vi "cd-maker.vi"() -> ()   [LabVIEW 2020]
uses:
  <vilib>/Utility/file.llb/Read Delimited Spreadsheet (I64).vi
  <vilib>/Utility/file.llb/Write Delimited Spreadsheet (DBL).vi
  <vilib>/express/express analysis/Spectral/Block/exnSpectralBlock spectral measurements power poly.vi
  <vilib>/express/express analysis/Spectral/Block/exnSpectralBlock spectral measurements power DDT.vi
  <vilib>/express/express analysis/Spectral/XNode/ExpressSpectralMeasurementsBlockNode.xnode
panel:
  in  "Timeout":i32
  out "Waveform Graph 2":dynamicdata(graph)
  out "Waveform Graph":dynamicdata(graph)
  in  "Добавлять точки при\nувеличении размера холста":bool=TRUE
  in  "Очистить полностью":bool
  in  "Стоп":bool
  in  "Путь для загрузки холста карты":path
  in  "Заполнить полностью":bool
  in  "Загрузить холст карты из файла":bool
  in  "Точки холста":bool[][](array[boolean])=[[FALSE, FALSE, FALSE, TRUE, FALSE, TRUE, FALSE, FALSE, FALSE], [FALSE, TRUE, FALSE, FALSE, FALSE, FALSE, FALSE, TRUE, FALSE], [FALSE, FALSE, FALSE, FALSE, FALSE, FALSE, FALSE, FALSE, FALSE], [TRUE, FALSE, FALSE, TRUE, FALSE, TRUE, FALSE, FALSE, TRUE], [FALSE, FALSE, FALSE, FALSE, FALSE, FALSE, FALSE, FALSE, FALSE], [TRUE, FALSE, FALSE, TRUE, FALSE, TRUE, FALSE, FALSE, TRUE], [FALSE, FALSE, FALSE, FALSE, FALSE, FALSE, FALSE, FALSE, FALSE], [FALSE, TRUE, FALSE, FALSE, FALSE, FALSE, FALSE, TRUE, FALSE], [FALSE, FALSE, FALSE, TRUE, FALSE, TRUE, FALSE, FALSE, FALSE]]
  out "Массив I и Q":cluster{"I":sgl, "Q":sgl}[](array[cluster])
  in  "I интервал":sgl=1.0 min=1 step=1
  in  "I смещение":sgl
  in  "Q интервал":sgl=1.0 min=1 step=1
  in  "Q смещение":sgl
  out "Карта":cluster{cluster{"I":sgl, "Q":sgl}[]}[](graph)=[{[{"I"=-1.0, "Q"=4.0}, {"I"=1.0, "Q"=4.0}, {"I"=-3.0, "Q"=3.0}, {"I"=3.0, "Q"=3.0}, {"I"=-4.0, "Q"=1.0}, {"I"=-1.0, "Q"=1.0}, {"I"=1.0, "Q"=1.0}, {"I"=4.0, "Q"=1.0}, {"I"=-4.0, "Q"=-1.0}, {"I"=-1.0, "Q"=-1.0}, {"I"=1.0, "Q"=-1.0}, {"I"=4.0, "Q"=-1.0}, {"I"=-3.0, "Q"=-3.0}, {"I"=3.0, "Q"=-3.0}, {"I"=-1.0, "Q"=-4.0}, {"I"=1.0, "Q"=-4.0}]}, {[{"I"=10.0, "Q"=0.0}, {"I"=-10.0, "Q"=0.0}, {"I"=0.0, "Q"=10.0}, {"I"=0.0, "Q"=-10.0}]}]
  in  "Размер холста":i32(slide)=4 min=1 max=30 step=1 scale=0.0..10.0
  in  "Путь для сохранения холста карты":path
  in  "Сохранить холст карты в файл":bool
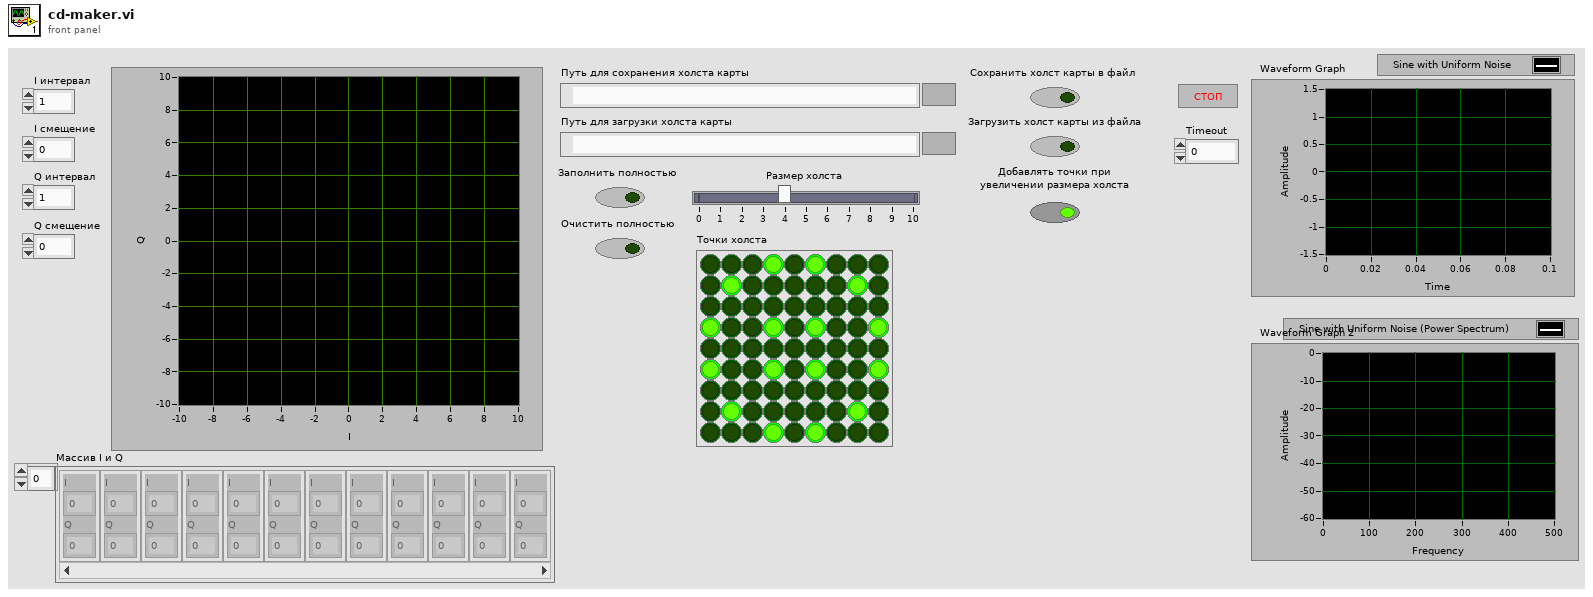
[diagram p1: front panel]
types:
  T1 = cluster{"averaging mode":u16, "weighting mode":u16, "number of averages":u32}
  T2 = cluster{"dB On (F)":bool, "unwrap phase (F)":bool, "convert to degree (F)":bool}
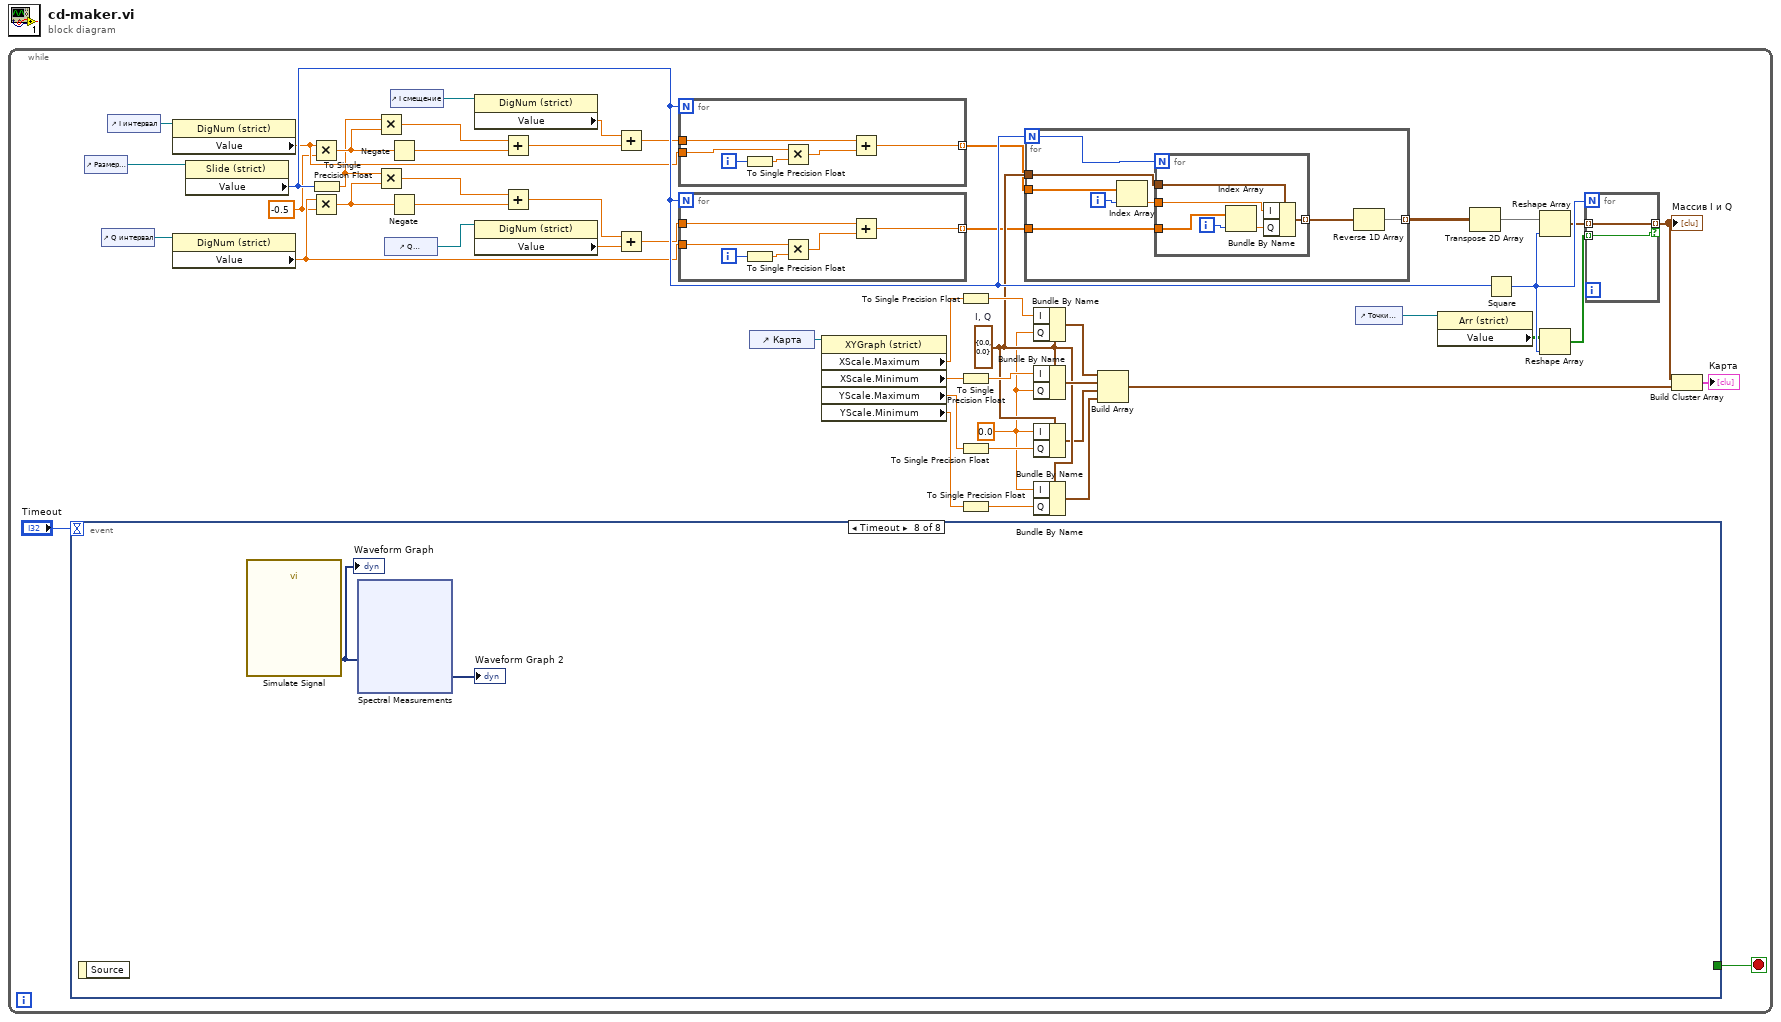
[diagram p0: block diagram]
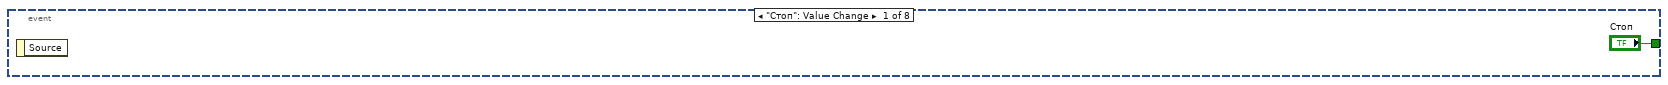
[diagram p2: hidden frame]
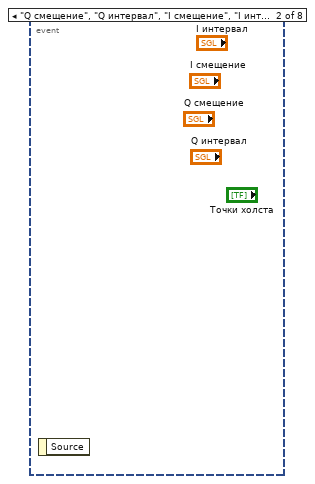
[diagram p3: hidden frame]
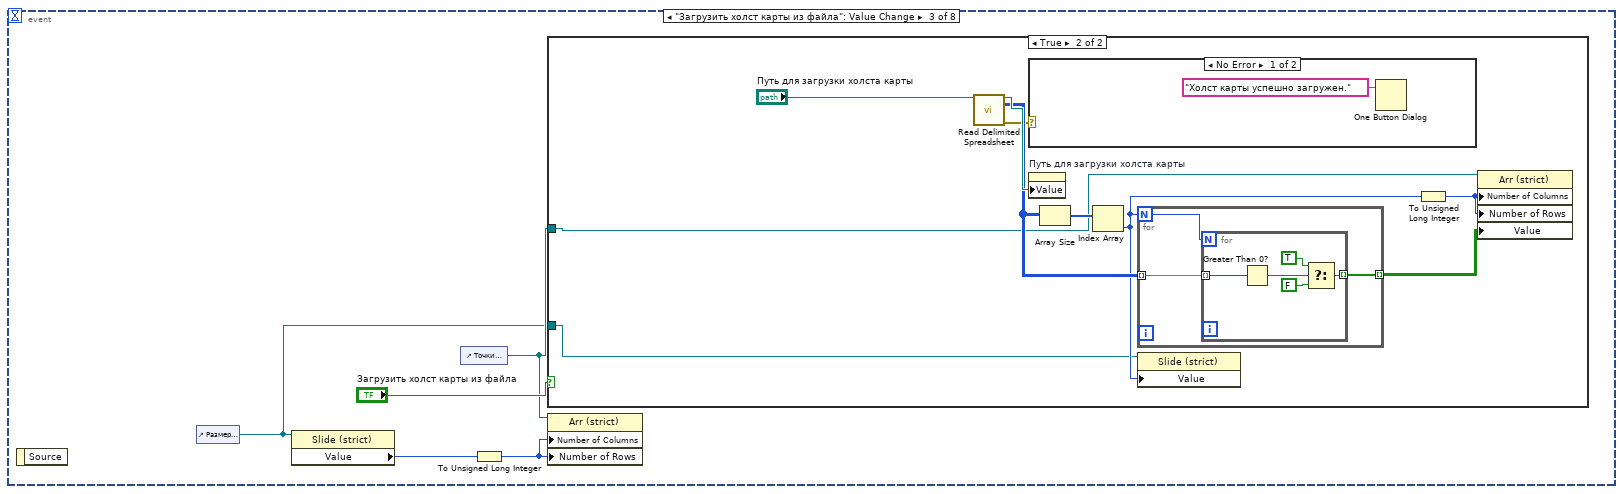
[diagram p4: hidden frame]
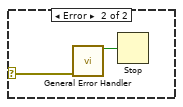
[diagram p6: hidden frame]
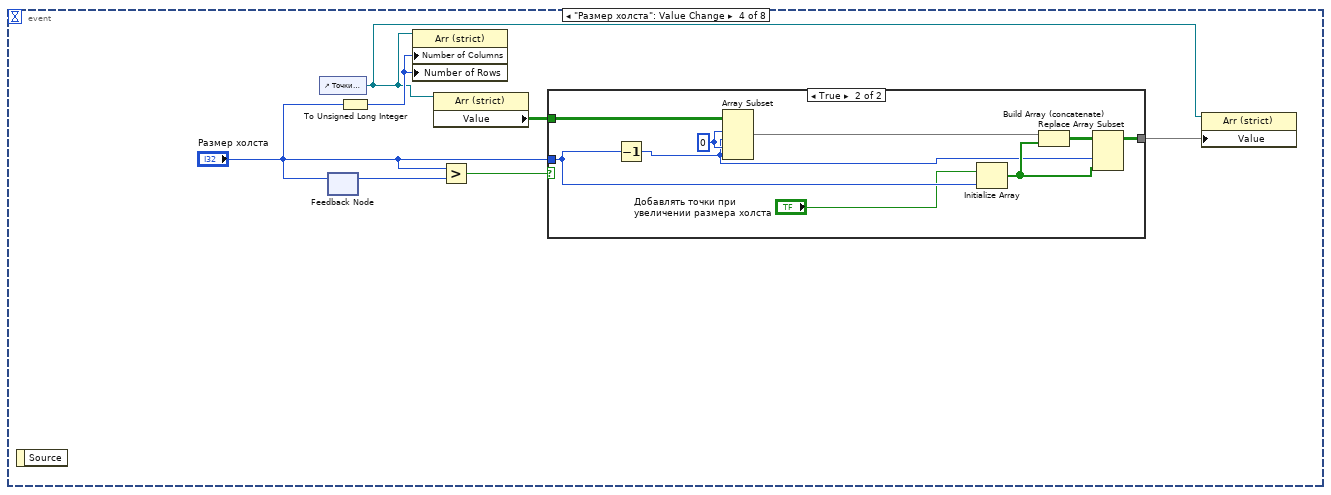
[diagram p7: hidden frame]
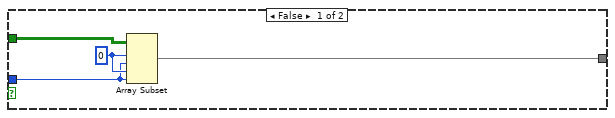
[diagram p8: hidden frame]
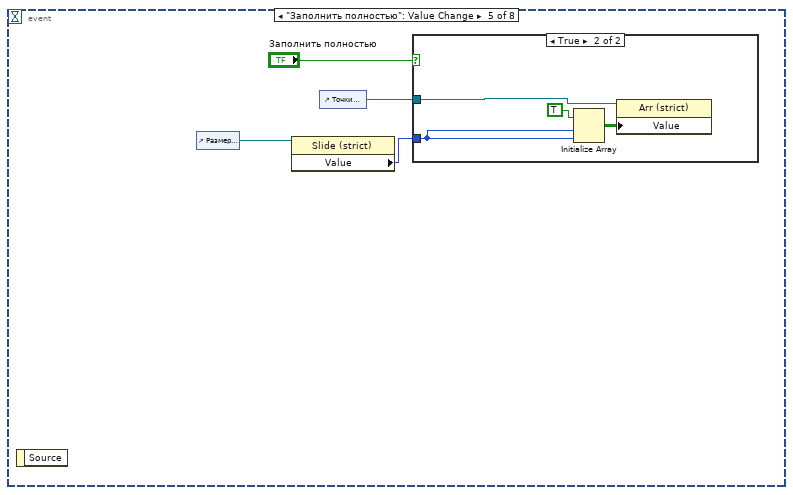
[diagram p9: hidden frame]
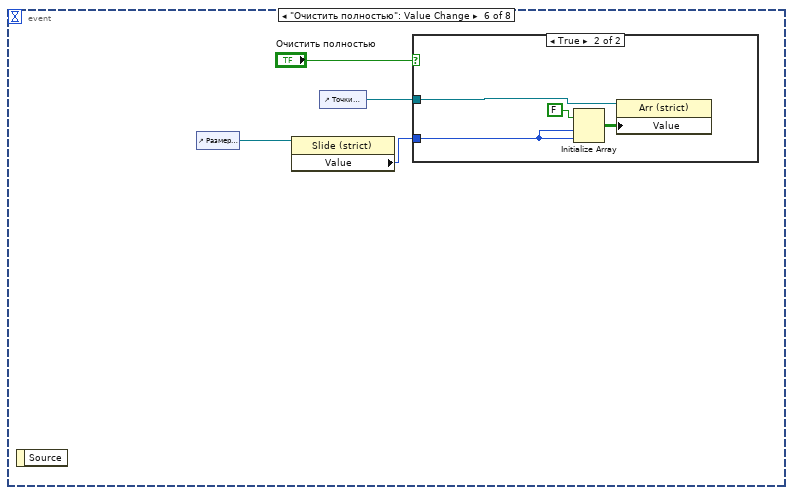
[diagram p11: hidden frame]
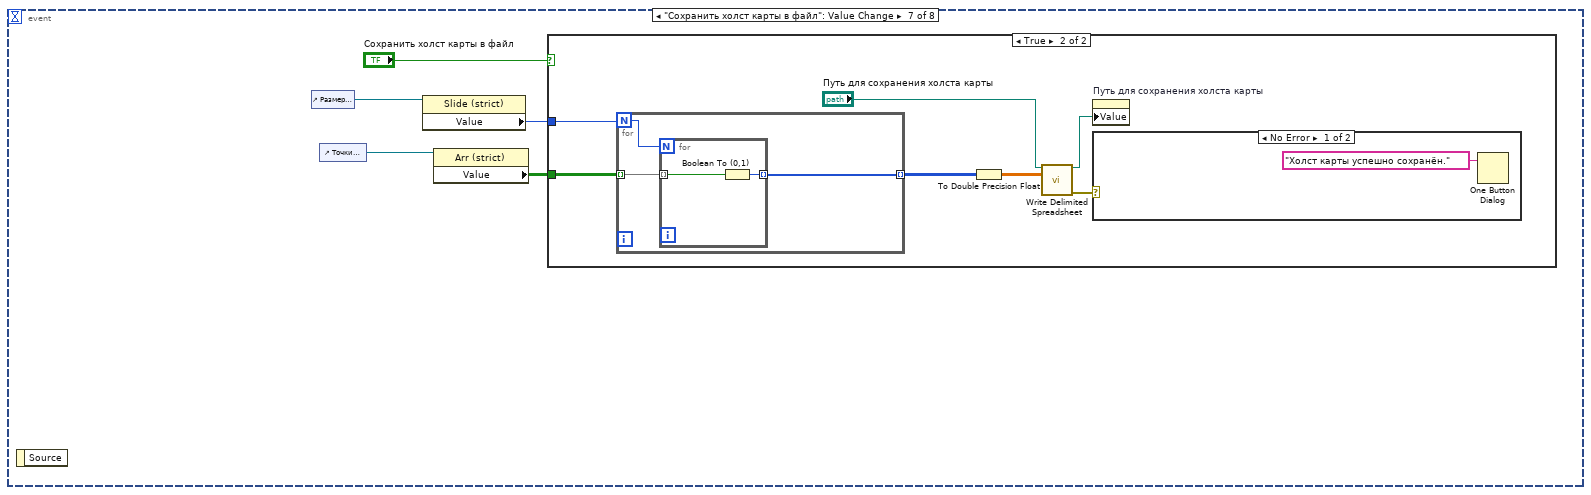
[diagram p13: hidden frame]
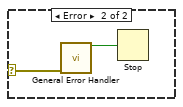
[diagram p15: hidden frame]
diagram:
  n1 = while {
    stop <- w46 stop-if-true
    w8 = sgl -0.5 ("y")
    w24 = sgl 0.0 ("Q")
    w27 = cluster{"I":sgl, "Q":sgl} {"I"=0.0, "Q"=0.0}  # I, Q
    n2 = event shown="[7] Timeout" {
      selector: _ -> [_ _ _ _ _ _ _ _]
      dyn-events: _ -> [_ _ _ _ _ _ _ _]
      timeout: "Timeout" -> [_ _ _ _ _ _ _ _]
      tunnel: ["Стоп" _ _ _ _ _ _ _] -> w46
      event "Стоп": Value Change {
        n3 = event-data() -> ()  [unwired: 1 in, 1 out]
      }
      event "Q смещение", "Q интервал", "I смещение", "I интервал", "Точки холста": Value Change {
        n4 = event-data() -> ()  [unwired: 1 in, 1 out]
      }
      event "Загрузить холст карты из файла": Value Change {
        n5 = event-data() -> ()  [unwired: 1 in, 1 out]
        n6 = control-ref of="Размер холста"() -> (w81:refnum<vi>)
        n7 = property class="Slide (strict)"(reference=w81) -> ("Value"=w84:i32)  [unwired: 1 in, 2 out]
        n8 = control-ref of="Точки холста"() -> (w82:refnum<vi>)
        n9 = To Unsigned Long Integer(number=w84) -> (unsigned 32bit integer=w83:u32)
        n10 = case shown="True" "Загрузить холст карты из файла" {
          tunnel: w82 -> [_ w88]
          tunnel: w81 -> [_ w86]
          frame False {
          }
          frame True {
            n11 = call-poly <vilib>:"Read Delimited Spreadsheet.vi"("file path (dialog if empty)"="Путь для загрузки холста карты") -> ("new file path (Not A Path if cancelled)"=w95:path, "all rows"=w92:i64[][], "error out"=w89:errorcluster)  [unwired: 9 in, 3 out]
            n12 = case shown="No Error" w89 {
              selector: w89 -> [_ w98]
              frame No Error {
                n13 = One Button Dialog(message="Холст карты успешно загружен.") -> ()  [unwired: 1 in, 1 out]
              }
              frame Error {
                n14 = call <vilib>:"General Error Handler.vi"("error in (no error)"=w98) -> ("error?"=w97:bool)  [unwired: 10 in, 4 out]
                n15 = Stop(stop? (T)=w97) -> ()
              }
            }
            n16 = property on="Путь для загрузки холста карты" class="Path"("Value"=w95) -> ()  [unwired: 2 in, 2 out]
            n17 = Array Size(array=w92) -> (size(s)=w93:i32[])
            n18 = Index Array(array=w93) -> (element=w87:i32)  [unwired: 1 in]
            n19 = for {
              N: w87 -> [w101]
              tunnel: w92 -> [w100] mode=indexing
              tunnel: [w99] -> w91 mode=indexing
              n20 = for {
                N: w101 -> [_]
                tunnel: w100 -> [w103] mode=indexing
                tunnel: [w104] -> w99 mode=indexing
                n21 = Greater Than 0?(x=w103) -> (x > 0?=w102:bool)
                n22 = Select(t=TRUE, s=w102, f=FALSE) -> (s? t:f=w104:bool)
              }
            }
            n23 = property class="Slide (strict)"(reference=w86, "Value"=w87) -> ()  [unwired: 1 in, 2 out]
            n24 = To Unsigned Long Integer(number=w87) -> (unsigned 32bit integer=w90:u32)
            n25 = property class="Arr (strict)"(reference=w88, "Number of Columns"=w90, "Number of Rows"=w90, "Value"=w91) -> ()  [unwired: 1 in, 2 out]
          }
        }
        n26 = property class="Arr (strict)"(reference=w82, "Number of Columns"=w83, "Number of Rows"=w83) -> ()  [unwired: 1 in, 2 out]
      }
      event "Размер холста": Value Change {
        n27 = event-data() -> ()  [unwired: 1 in, 1 out]
        n28 = control-ref of="Точки холста"() -> (w108:refnum<vi>)
        n29 = feedback #1() -> (w107:i32)  [unwired: 1 in]
        n30 = feedback-in #1("Размер холста") -> ()
        n31 = To Unsigned Long Integer(number="Размер холста") -> (unsigned 32bit integer=w113:u32)
        n32 = property class="Arr (strict)"(reference=w108, "Number of Columns"=w113, "Number of Rows"=w113) -> ()  [unwired: 1 in, 2 out]
        n33 = property class="Arr (strict)"(reference=w108) -> ("Value"=w111:bool[][])  [unwired: 1 in, 2 out]
        n34 = Greater?(x="Размер холста", y=w107) -> (0:w110:bool)
        n35 = case shown="True" w110 {
          tunnel: "Размер холста" -> [w115 w119]
          tunnel: w111 -> [w116 w125]
          tunnel: [w114 w123] -> w112
          frame False {
            w117 = 0 ("index")
            n36 = Array Subset(array=w116, index (row)=w117, length (row)=w115, index (col)=w117, length (col)=w115) -> (w114:bool[][])
          }
          frame True {
            w126 = 0 ("index")
            n37 = Decrement(x=w119) -> (x-1=w120:i32)
            n38 = Array Subset(array=w125, index (row)=w126, length (row)=w120, index (col)=w126, length (col)=w120) -> (w124:bool[][])
            n39 = Initialize Array("Добавлять точки при\nувеличении размера холста", w119) -> (w122:bool[])
            n40 = Build Array (concatenate)(w124, w122) -> (w121:bool[][])
            n41 = Replace Array Subset(array=w121, new element=w122, index (col)=w120) -> (w123:bool[][])  [unwired: 1 in]
          }
        }
        n42 = property class="Arr (strict)"(reference=w108, "Value"=w112) -> ()  [unwired: 1 in, 2 out]
      }
      event "Заполнить полностью": Value Change {
        n43 = event-data() -> ()  [unwired: 1 in, 1 out]
        n44 = control-ref of="Размер холста"() -> (w128:refnum<vi>)
        n45 = property class="Slide (strict)"(reference=w128) -> ("Value"=w127:i32)  [unwired: 1 in, 2 out]
        n46 = control-ref of="Точки холста"() -> (w129:refnum<vi>)
        n47 = case shown="True" "Заполнить полностью" {
          tunnel: w129 -> [_ w132]
          tunnel: w127 -> [_ w131]
          frame False {
          }
          frame True {
            n48 = Initialize Array(TRUE, w131, w131) -> (w133:bool[][])
            n49 = property class="Arr (strict)"(reference=w132, "Value"=w133) -> ()  [unwired: 1 in, 2 out]
          }
        }
      }
      event "Очистить полностью": Value Change {
        n50 = event-data() -> ()  [unwired: 1 in, 1 out]
        n51 = control-ref of="Размер холста"() -> (w136:refnum<vi>)
        n52 = property class="Slide (strict)"(reference=w136) -> ("Value"=w135:i32)  [unwired: 1 in, 2 out]
        n53 = control-ref of="Точки холста"() -> (w137:refnum<vi>)
        n54 = case shown="True" "Очистить полностью" {
          tunnel: w137 -> [_ w140]
          tunnel: w135 -> [_ w139]
          frame False {
          }
          frame True {
            n55 = Initialize Array(FALSE, w139, w139) -> (w141:bool[][])
            n56 = property class="Arr (strict)"(reference=w140, "Value"=w141) -> ()  [unwired: 1 in, 2 out]
          }
        }
      }
      event "Сохранить холст карты в файл": Value Change {
        n57 = event-data() -> ()  [unwired: 1 in, 1 out]
        n58 = control-ref of="Размер холста"() -> (w144:refnum<vi>)
        n59 = control-ref of="Точки холста"() -> (w146:refnum<vi>)
        n60 = property class="Slide (strict)"(reference=w144) -> ("Value"=w143:i32)  [unwired: 1 in, 2 out]
        n61 = property class="Arr (strict)"(reference=w146) -> ("Value"=w145:bool[][])  [unwired: 1 in, 2 out]
        n62 = case shown="True" "Сохранить холст карты в файл" {
          tunnel: w143 -> [_ w149]
          tunnel: w145 -> [_ w148]
          frame False {
          }
          frame True {
            n63 = for {
              N: w149 -> [w155]
              tunnel: w148 -> [w157] mode=indexing
              tunnel: [w156] -> w151 mode=indexing
              n64 = for {
                N: w155 -> [_]
                tunnel: w157 -> [w158] mode=indexing
                tunnel: [w159] -> w156 mode=indexing
                n65 = Boolean To (0,1)(Boolean=w158) -> (0, 1=w159:i16)
              }
            }
            n66 = To Double Precision Float(number=w151) -> (double precision float=w152:dbl[][])
            n67 = call-poly <vilib>:"Write Delimited Spreadsheet.vi"("file path (dialog if empty)"="Путь для сохранения холста карты", "2D data"=w152) -> ("new file path (Not A Path if cancelled)"=w150:path, "error out"=w153:errorcluster)  [unwired: 12 in]
            n68 = property on="Путь для сохранения холста карты" class="Path"("Value"=w150) -> ()  [unwired: 2 in, 2 out]
            n69 = case shown="No Error" w153 {
              selector: w153 -> [_ w162]
              frame No Error {
                n70 = One Button Dialog(message="Холст карты успешно сохранён.") -> ()  [unwired: 1 in, 1 out]
              }
              frame Error {
                n71 = call <vilib>:"General Error Handler.vi"("error in (no error)"=w162) -> ("error?"=w161:bool)  [unwired: 10 in, 4 out]
                n72 = Stop(stop? (T)=w161) -> ()
              }
            }
          }
        }
      }
      event Timeout {
        n73 = event-data() -> ()  [unwired: 1 in, 1 out]
        n74 = call "Simulate Signal"() -> ("Sine with Uniform Noise"=w164:dynamicdata)  [unwired: 14 in, 1 out]
        "Waveform Graph" <- w164
        n75 = xnode "Spectral Measurements"("Signals"=w164) -> ("Power Spectrum"=→"Waveform Graph 2":dynamicdata)  [unwired: 1 in, 1 out]
      }
    }
    n76 = control-ref of="Размер холста"() -> (w43:refnum<vi>)
    n77 = control-ref of="Q интервал"() -> (w39:refnum<vi>)
    n78 = control-ref of="I интервал"() -> (w41:refnum<vi>)
    n79 = property class="DigNum (strict)"(reference=w41) -> ("Value"=w12:sgl)  [unwired: 1 in, 2 out]
    n80 = property class="DigNum (strict)"(reference=w39) -> ("Value"=w9:sgl)  [unwired: 1 in, 2 out]
    n81 = property class="Slide (strict)"(reference=w43) -> ("Value"=w42:i32)  [unwired: 1 in, 2 out]
    n82 = Multiply(x=w12, y=w8) -> (x*y=w11:sgl)
    n83 = Multiply(x=w9, y=w8) -> (x*y=w6:sgl)
    n84 = To Single Precision Float(number=w42) -> (single precision float=w10:sgl)
    n85 = Multiply(x=w10, y=w11) -> (x*y=w18:sgl)
    n86 = Multiply(x=w10, y=w6) -> (x*y=w7:sgl)
    n87 = control-ref of="Q смещение"() -> (w38:refnum<vi>)
    n88 = Negate(x=w11) -> (-x=w13:sgl)
    n89 = Negate(x=w6) -> (-x=w5:sgl)
    n90 = control-ref of="I смещение"() -> (w40:refnum<vi>)
    n91 = property class="DigNum (strict)"(reference=w40) -> ("Value"=w37:sgl)  [unwired: 1 in, 2 out]
    n92 = property class="DigNum (strict)"(reference=w38) -> ("Value"=w16:sgl)  [unwired: 1 in, 2 out]
    n93 = Add(x=w18, y=w13) -> (x+y=w14:sgl)
    n94 = Add(x=w7, y=w5) -> (x+y=w4:sgl)
    n95 = Add(x=w37, y=w14) -> (x+y=w15:sgl)
    n96 = Add(x=w4, y=w16) -> (x+y=w17:sgl)
    n97 = for {
      N: w42 -> [_]
      tunnel: [w74] -> w3 mode=indexing
      tunnel: w12 -> [w75]
      tunnel: w15 -> [w76]
      i -> [w77]
      n98 = To Single Precision Float(number=w77) -> (single precision float=w78:sgl)
      n99 = Multiply(x=w75, y=w78) -> (x*y=w79:sgl)
      n100 = Add(x=w76, y=w79) -> (x+y=w74:sgl)
    }
    n101 = for {
      N: w42 -> [_]
      tunnel: [w54] -> w2 mode=indexing
      tunnel: w9 -> [w56]
      tunnel: w17 -> [w58]
      i -> [w55]
      n102 = To Single Precision Float(number=w55) -> (single precision float=w59:sgl)
      n103 = Multiply(x=w56, y=w59) -> (x*y=w57:sgl)
      n104 = Add(x=w58, y=w57) -> (x+y=w54:sgl)
    }
    n105 = control-ref of="Карта"() -> (w36:refnum<vi>)
    n106 = property class="XYGraph (strict)"(reference=w36) -> ("XScale.Maximum"=w35:dbl, "XScale.Minimum"=w34:dbl, "YScale.Maximum"=w33:dbl, "YScale.Minimum"=w32:dbl)  [unwired: 1 in, 2 out]
    n107 = To Single Precision Float(number=w35) -> (single precision float=w31:sgl)
    n108 = To Single Precision Float(number=w34) -> (single precision float=w30:sgl)
    n109 = To Single Precision Float(number=w33) -> (single precision float=w26:sgl)
    n110 = To Single Precision Float(number=w32) -> (single precision float=w25:sgl)
    n111 = for {
      N: w42 -> [w64]
      tunnel: w2 -> [w65]
      tunnel: [w61] -> w51 mode=indexing
      tunnel: w3 -> [w63]
      tunnel: w27 -> [w60]
      i -> [w66]
      n112 = Index Array ("Index values")(array=w63, index=w66) -> (element=w67:sgl)
      n113 = for {
        N: w64 -> [_]
        tunnel: w67 -> [w71]
        tunnel: w65 -> [w72]
        tunnel: [w69] -> w62 mode=indexing
        tunnel: w60 -> [w68]
        i -> [w73]
        n114 = Index Array(array=w72, index=w73) -> (element=w70:sgl)
        n115 = Bundle By Name(cluster=w68, "I"=w71, "Q"=w70) -> (w69:cluster{"I":sgl, "Q":sgl})
      }
      n116 = Reverse 1D Array(array=w62) -> (reversed array=w61:cluster{"I":sgl, "Q":sgl}[])
    }
    n117 = Bundle By Name(cluster=w27, "I"=w31, "Q"=w24) -> (w29:cluster{"I":sgl, "Q":sgl})
    n118 = Bundle By Name(cluster=w27, "I"=w30, "Q"=w24) -> (w28:cluster{"I":sgl, "Q":sgl})
    n119 = Bundle By Name(cluster=w27, "I"=w24, "Q"=w26) -> (w23:cluster{"I":sgl, "Q":sgl})
    n120 = Bundle By Name(cluster=w27, "I"=w24, "Q"=w25) -> (w22:cluster{"I":sgl, "Q":sgl})
    n121 = Build Array(w29, w28, w23, w22) -> (w20:cluster{"I":sgl, "Q":sgl}[])
    n122 = control-ref of="Точки холста"() -> (w45:refnum<vi>)
    n123 = property class="Arr (strict)"(reference=w45) -> ("Value"=w44:bool[][])  [unwired: 1 in, 2 out]
    n124 = Transpose 2D Array(2D array=w51) -> (transposed array=w50:cluster{"I":sgl, "Q":sgl}[][])
    n125 = Square(x=w42) -> (x^2=w49:i32)
    n126 = Reshape Array(w50, w49) -> (w48:cluster{"I":sgl, "Q":sgl}[])
    n127 = Reshape Array(w44, w49) -> (w47:bool[])
    n128 = for {
      N: w49 -> [_]
      tunnel: w48 -> [w53] mode=indexing
      tunnel: [w53] -> w21 mode=indexing if=w52
      tunnel: w47 -> [w52] mode=indexing
    }
    "Массив I и Q" <- w21
    n129 = Build Cluster Array(w21, w20) -> (→"Карта":cluster{cluster{"I":sgl, "Q":sgl}[]}[])
  }
